vi "6221_arb_waveform.vi"(0 "Waveform Input":T1={"Initial Value"=0.0, "Final Value"=0.0, "Tau"=0.0, "Eta"=0.0, "Nickname"="Channel 0 D", "Function Type"=enum."Power Law", "Conversion"=enum."Volts", "Constant"=0.0}, 2 "Phase Time":dbl, 3 "Sample Rate":dbl) -> (7 "Waveform Output":T1={"Initial Value"=0.0, "Final Value"=0.0, "Tau"=0.0, "Eta"=0.0, "Nickname"="Channel 0 D", "Function Type"=enum."Power Law", "Conversion"=enum."Volts", "Constant"=0.0}, 8 "output waveform":waveform(dbl), 9 "# Samples":dbl)   [LabVIEW 2016]
uses:
  6221_waveform_param.ctl
  6733_Red_MOT/Neutral_voltage_conversion_control.ctl
panel:
  out "beta":dbl
  out "dt":dbl
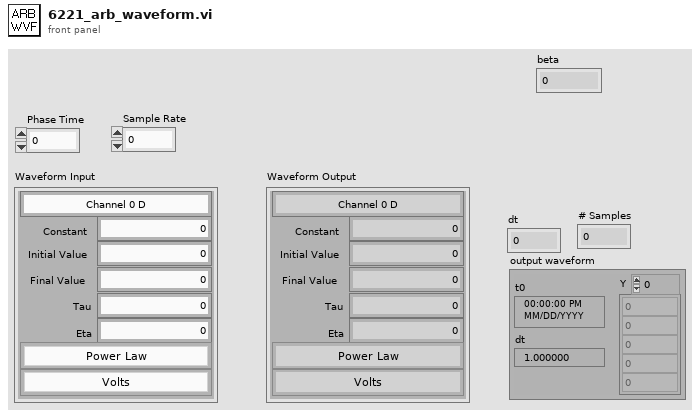
[diagram p1: front panel]
types:
  T1 = typedef "6221_waveform_param.ctl" = cluster{"Initial Value":dbl, "Final Value":dbl, "Tau":dbl, "Eta":dbl, "Nickname":string, "Function Type":enum16{"Constant", "Power Law", "Evap - Calc Tau", "Evaporation Formula", "Tanh", "Exponential"}, "Conversion":T2, "Constant":dbl}
  T2 = typedef "Neutral_voltage_conversion_control.ctl" = enum16{"Volts", "B Field Grad (G/cm)", "Red Boson Cntr Freq (MHz)", "Red Boson Dither Amp (kHz)", "Red Boson Power (mW)", "Red 87 Trap Cntr Freq (MHz)", "Red 87 Trap Dither Amp (kHz)", "Red 87 Trap Power (mW)", "Red 87 Stir Cntr Freq (MHz)", "Red 87 Stir Dither Amp (kHz)", "Red 87 Stir Power (mW)", "ODT Sheet Trap Power (W)", "ODT Loading Trap Power (W)"}
  T3 = enum16{"Constant", "Power Law", "Evap - Calc Tau", "Evaporation Formula", "Tanh", "Exponential"}
  T4 = cluster{"Initial Value":dbl, "Final Value":dbl, "Tau":dbl, "Eta":dbl, "Nickname":string, "Function Type":enum16{"Constant", "Power Law", "Evap - Calc Tau", "Evaporation Formula", "Tanh", "Exponential"}, "Conversion":T2, "Constant":dbl}
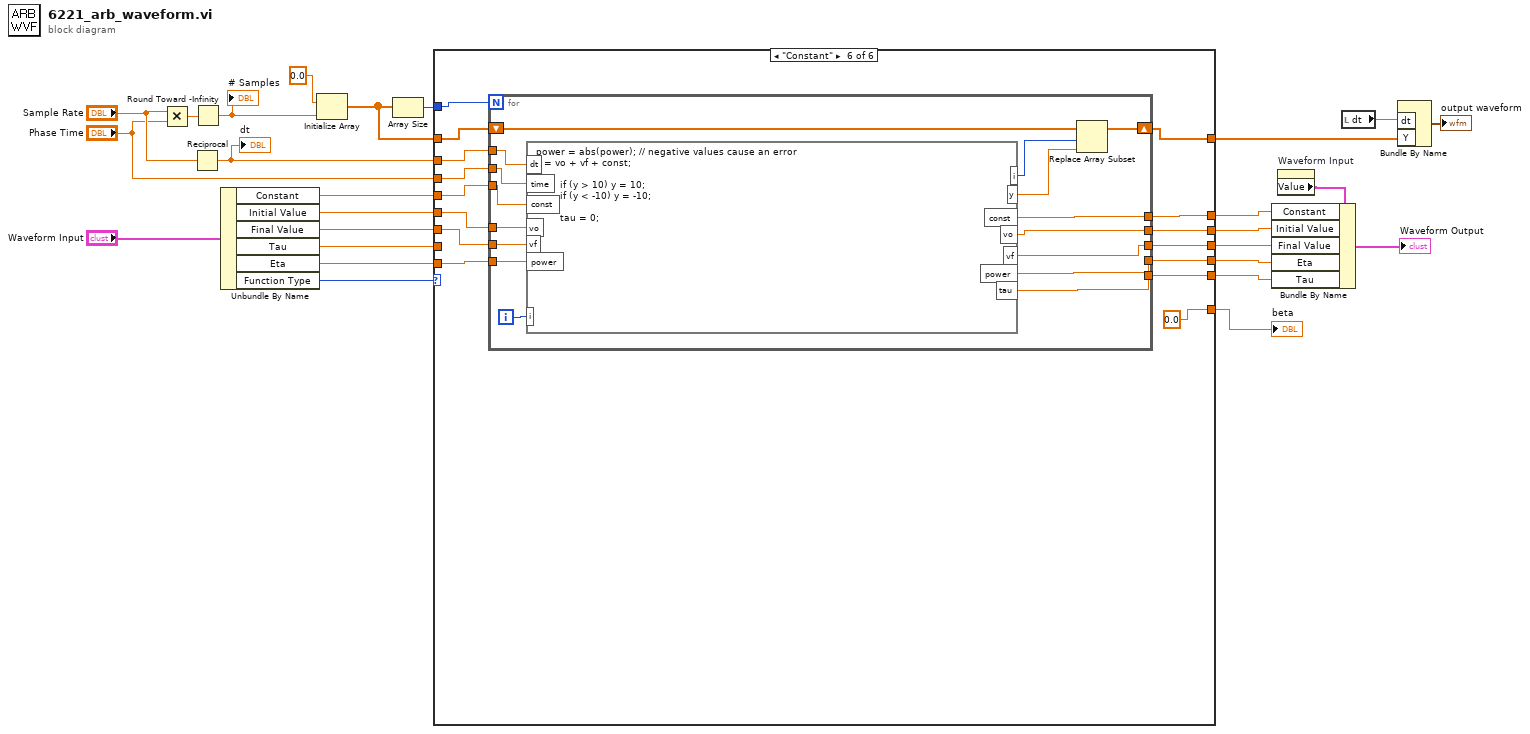
[diagram p0: block diagram]
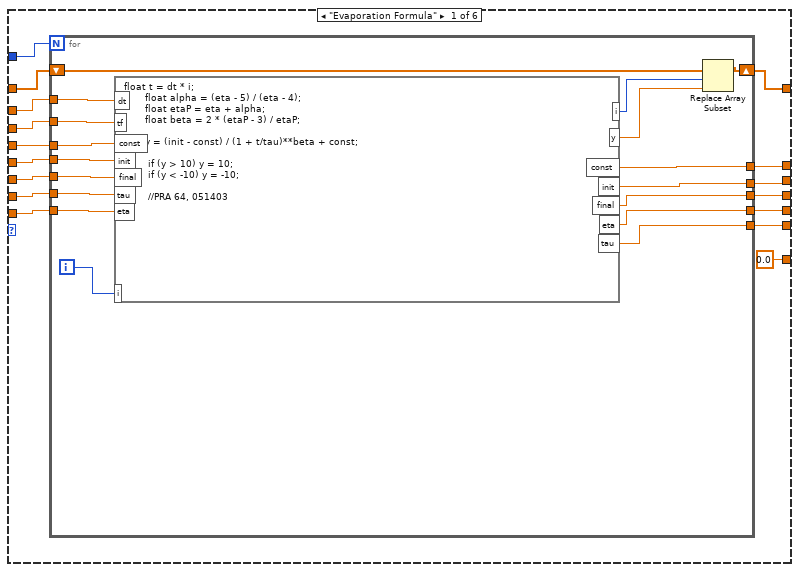
[diagram p2: hidden frame]
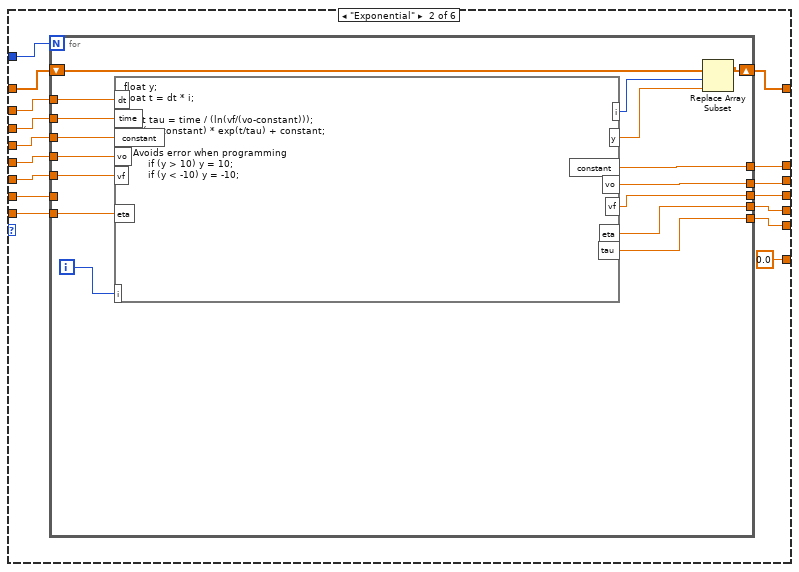
[diagram p3: hidden frame]
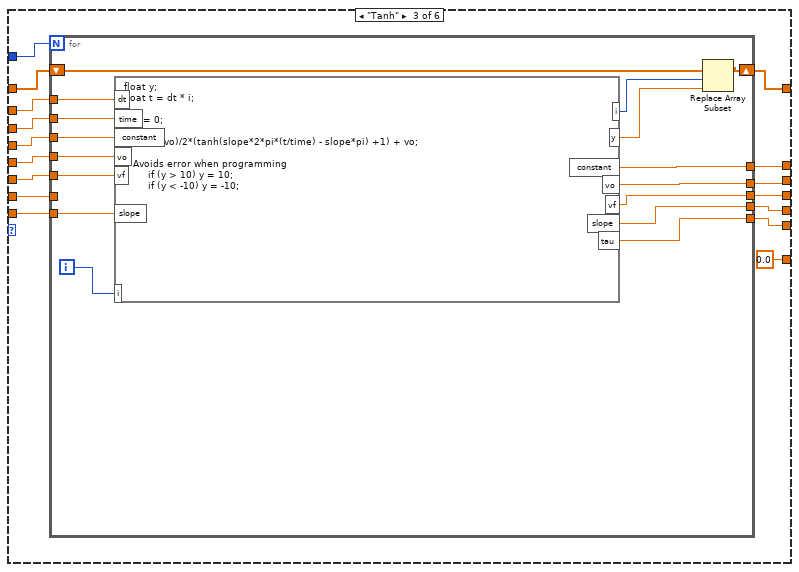
[diagram p4: hidden frame]
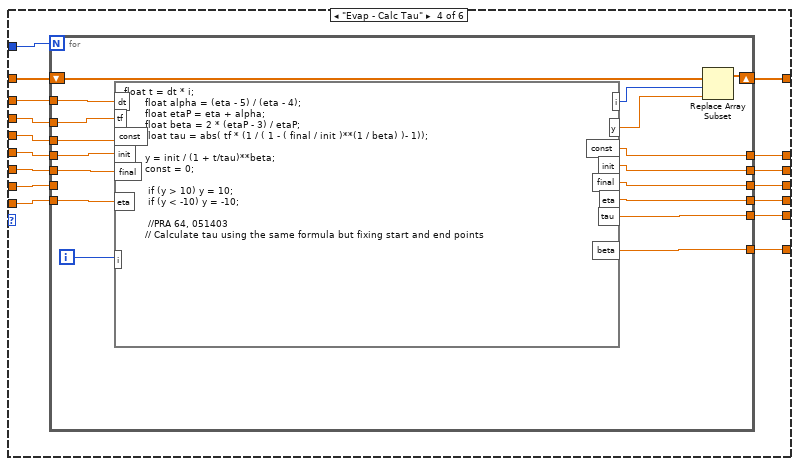
[diagram p5: hidden frame]
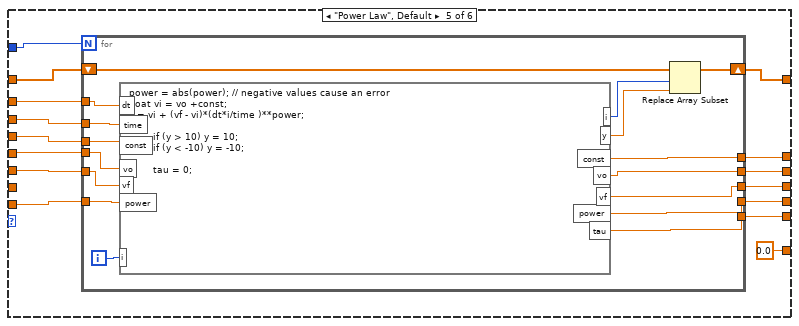
[diagram p6: hidden frame]
diagram:
  n1 = Multiply(x="Sample Rate", y="Phase Time") -> (x*y=w3:dbl)
  n2 = Reciprocal(x="Sample Rate") -> (1/x=w17:dbl)
  "dt" <- w17
  n3 = Round Toward -Infinity(1:w3) -> (0:w2:dbl)
  "# Samples" <- w2
  n4 = Unbundle By Name("Waveform Input") -> ("Constant"=w11:dbl, "Initial Value"=w21:dbl, "Final Value"=w22:dbl, "Tau"=w23:dbl, "Eta"=w24:dbl, "Function Type"=w26:T3)
  n5 = Initialize Array(0.0 ("element"), w2) -> (w18:dbl[])
  n6 = Array Size(array=w18) -> (size(s)=w19:i32)
  n7 = case shown="\"Constant\"" w26 {
    tunnel: w24 -> [w36 w69 w101 w133 w169 w196]
    tunnel: w23 -> [w37 w70 w102 w134 _ _]
    tunnel: w22 -> [w38 w71 w103 w135 w170 w195]
    tunnel: w21 -> [w39 w72 w104 w136 w171 w194]
    tunnel: w19 -> [w42 w75 w107 w139 w164 w188]
    tunnel: w18 -> [w41 w74 w106 w138 w166 w190]
    tunnel: w17 -> [w40 w73 w105 w137 w167 w191]
    tunnel: [w35 w68 w100 w132 w165 w189] -> w16
    tunnel: "Phase Time" -> [w34 w67 w99 w131 w168 w192]
    tunnel: w11 -> [w33 w66 w98 w130 w163 w193]
    tunnel: [w31 w64 w96 w129 w162 w202] -> w10
    tunnel: [w30 w63 w95 w128 w160 w201] -> w9
    tunnel: [w32 w65 w97 w127 w161 w200] -> w8
    tunnel: [w29 w62 w94 w126 w159 w199] -> w7
    tunnel: [w28 w61 w93 w125 w158 w198] -> w6
    tunnel: [0.0 0.0 0.0 w124 0.0 0.0] -> w5
    frame "Evaporation Formula" {
      n8 = for {
        N: w42 -> [_]
        shift-right: [w51] -> w35
        shift-left: w41 -> [w53]
        tunnel: w40 -> [w58]
        tunnel: w39 -> [w55]
        tunnel: w38 -> [w56]
        tunnel: w37 -> [w57]
        tunnel: w36 -> [w59]
        tunnel: w34 -> [w50]
        tunnel: w33 -> [w49]
        tunnel: [w43] -> w32
        tunnel: [w47] -> w31
        tunnel: [w46] -> w30
        tunnel: [w45] -> w29
        tunnel: [w44] -> w28
        i -> [w54]
        n9 = formula code="float t = dt * i;\n       float alpha = (eta - 5) / (eta - 4);\n       float etaP = eta + alpha;\n       float beta = 2 * (etaP - 3) / etaP;\n\n       y = (init - const) / (1 + t/tau)**beta + const;\n\n        if (y > 10) y = 10;\n        if (y < -10) y = -10;\n\n        //PRA 64, 051403"("eta"=w59, "tau"=w57, "init"=w55, "final"=w56, "i"=w54, "dt"=w58, "tf"=w50, "const"=w49) -> ("y"=w48:dbl, "i"=w52:i32, "const"=w47:dbl, "init"=w46:dbl, "eta"=w45:dbl, "tau"=w44:dbl, "final"=w43:dbl)
        n10 = Replace Array Subset(array=w53, new element=w48, index=w52) -> (w51:dbl[])
      }
    }
    frame "Exponential" {
      n11 = for {
        N: w75 -> [_]
        shift-right: [w84] -> w68
        shift-left: w74 -> [w86]
        tunnel: w73 -> [w90]
        tunnel: w72 -> [w88]
        tunnel: w71 -> [w89]
        tunnel: w70 -> [_]
        tunnel: w69 -> [w91]
        tunnel: w67 -> [w83]
        tunnel: w66 -> [w82]
        tunnel: [w76] -> w65
        tunnel: [w80] -> w64
        tunnel: [w79] -> w63
        tunnel: [w78] -> w62
        tunnel: [w77] -> w61
        i -> [w87]
        n12 = formula code="float y;\nfloat t = dt * i;\n\nfloat tau = time / (ln(vf/(vo-constant)));\ny = (vo-constant) * exp(t/tau) + constant;\n\n// Avoids error when programming\n        if (y > 10) y = 10;\n        if (y < -10) y = -10;"("eta"=w91, "vo"=w88, "vf"=w89, "i"=w87, "dt"=w90, "time"=w83, "constant"=w82) -> ("y"=w81:dbl, "i"=w85:i32, "constant"=w80:dbl, "vo"=w79:dbl, "eta"=w78:dbl, "tau"=w77:dbl, "vf"=w76:dbl)
        n13 = Replace Array Subset(array=w86, new element=w81, index=w85) -> (w84:dbl[])
      }
    }
    frame "Tanh" {
      n14 = for {
        N: w107 -> [_]
        shift-right: [w116] -> w100
        shift-left: w106 -> [w118]
        tunnel: w105 -> [w122]
        tunnel: w104 -> [w120]
        tunnel: w103 -> [w121]
        tunnel: w102 -> [_]
        tunnel: w101 -> [w123]
        tunnel: w99 -> [w115]
        tunnel: w98 -> [w114]
        tunnel: [w108] -> w97
        tunnel: [w112] -> w96
        tunnel: [w111] -> w95
        tunnel: [w110] -> w94
        tunnel: [w109] -> w93
        i -> [w119]
        n15 = formula code="float y;\nfloat t = dt * i;\n\ntau = 0;\n\ny = (vf - vo)/2*(tanh(slope*2*pi*(t/time) - slope*pi) +1) + vo;\n\n// Avoids error when programming\n        if (y > 10) y = 10;\n        if (y < -10) y = -10;"("slope"=w123, "vo"=w120, "vf"=w121, "i"=w119, "dt"=w122, "time"=w115, "constant"=w114) -> ("y"=w113:dbl, "i"=w117:i32, "constant"=w112:dbl, "vo"=w111:dbl, "slope"=w110:dbl, "tau"=w109:dbl, "vf"=w108:dbl)
        n16 = Replace Array Subset(array=w118, new element=w113, index=w117) -> (w116:dbl[])
      }
    }
    frame "Evap - Calc Tau" {
      n17 = for {
        N: w139 -> [_]
        shift-right: [w148] -> w132
        shift-left: w138 -> [w151]
        tunnel: w137 -> [w155]
        tunnel: w136 -> [w153]
        tunnel: w135 -> [w154]
        tunnel: w134 -> [_]
        tunnel: w133 -> [w156]
        tunnel: w131 -> [w147]
        tunnel: w130 -> [w146]
        tunnel: [w145] -> w129
        tunnel: [w144] -> w128
        tunnel: [w143] -> w127
        tunnel: [w142] -> w126
        tunnel: [w141] -> w125
        tunnel: [w140] -> w124
        i -> [w152]
        n18 = formula code="float t = dt * i;\n       float alpha = (eta - 5) / (eta - 4);\n       float etaP = eta + alpha;\n       float beta = 2 * (etaP - 3) / etaP;\n       float tau = abs( tf * (1 / ( 1 - ( final / init )**(1 / beta) )- 1));\n\n       y = init / (1 + t/tau)**beta;\n       const = 0;\n\n        if (y > 10) y = 10;\n        if (y < -10) y = -10;\n\n        //PRA 64, 051403\n       // Calculate tau using the same formula but fixing start and end points"("eta"=w156, "init"=w153, "final"=w154, "i"=w152, "dt"=w155, "tf"=w147, "const"=w146) -> ("y"=w149:dbl, "i"=w150:i32, "const"=w145:dbl, "init"=w144:dbl, "final"=w143:dbl, "eta"=w142:dbl, "tau"=w141:dbl, "beta"=w140:dbl)
        n19 = Replace Array Subset(array=w151, new element=w149, index=w150) -> (w148:dbl[])
      }
    }
    frame "Power Law", Default {
      n20 = for {
        N: w164 -> [_]
        tunnel: w171 -> [w187]
        tunnel: w170 -> [w186]
        tunnel: w169 -> [w185]
        tunnel: w168 -> [w184]
        tunnel: w167 -> [w183]
        shift-right: [w181] -> w165
        shift-left: w166 -> [w182]
        tunnel: w163 -> [w178]
        tunnel: [w177] -> w162
        tunnel: [w172] -> w161
        tunnel: [w175] -> w160
        tunnel: [w173] -> w159
        tunnel: [w174] -> w158
        i -> [w180]
        n21 = formula code="power = abs(power); // negative values cause an error\nfloat vi = vo +const;\ny = vi + (vf - vi)*(dt*i/time )**power;\n\n        if (y > 10) y = 10;\n        if (y < -10) y = -10;\n\n        tau = 0;"("vo"=w187, "vf"=w186, "time"=w184, "power"=w185, "i"=w180, "dt"=w183, "const"=w178) -> ("y"=w176:dbl, "i"=w179:i32, "const"=w177:dbl, "vo"=w175:dbl, "power"=w173:dbl, "tau"=w174:dbl, "vf"=w172:dbl)
        n22 = Replace Array Subset(array=w182, new element=w176, index=w179) -> (w181:dbl[])
      }
    }
    frame "Constant" {
      n23 = for {
        N: w188 -> [_]
        shift-right: [w217] -> w189
        shift-left: w190 -> [w218]
        tunnel: [w214] -> w202
        tunnel: [w203] -> w200
        tunnel: [w212] -> w201
        tunnel: [w211] -> w199
        tunnel: [w210] -> w198
        tunnel: w196 -> [w209]
        tunnel: w195 -> [w208]
        tunnel: w194 -> [w207]
        tunnel: w193 -> [w206]
        tunnel: w192 -> [w205]
        tunnel: w191 -> [w204]
        i -> [w216]
        n24 = formula code="power = abs(power); // negative values cause an error\ny = vo + vf + const;\n\n        if (y > 10) y = 10;\n        if (y < -10) y = -10;\n\n        tau = 0;"("vo"=w207, "vf"=w208, "time"=w205, "power"=w209, "i"=w216, "dt"=w204, "const"=w206) -> ("y"=w213:dbl, "i"=w215:i32, "const"=w214:dbl, "vo"=w212:dbl, "power"=w211:dbl, "tau"=w210:dbl, "vf"=w203:dbl)
        n25 = Replace Array Subset(array=w218, new element=w213, index=w215) -> (w217:dbl[])
      }
    }
  }
  "beta" <- w5
  n26 = property on="Waveform Input" class="Clust (strict)"() -> ("Value"=w4:T4)  [unwired: 2 in, 2 out]
  n27 = Bundle By Name(cluster=w4, "Constant"=w10, "Initial Value"=w9, "Final Value"=w8, "Eta"=w7, "Tau"=w6) -> (→"Waveform Output":T4)
  n28 = local read "dt"() -> (w15:dbl)
  n29 = Bundle By Name("dt"=w15, "Y"=w16) -> (→"output waveform":waveform(dbl))  [unwired: 1 in]
